vi "Test Parse State.vi"() -> ()   [LabVIEW 2020]
uses:
  <vilib>/regexp/Match Regular Expression.xnode
panel:
  out "Array 2":T1(array[cluster])
  out "Array":T1(array[cluster])
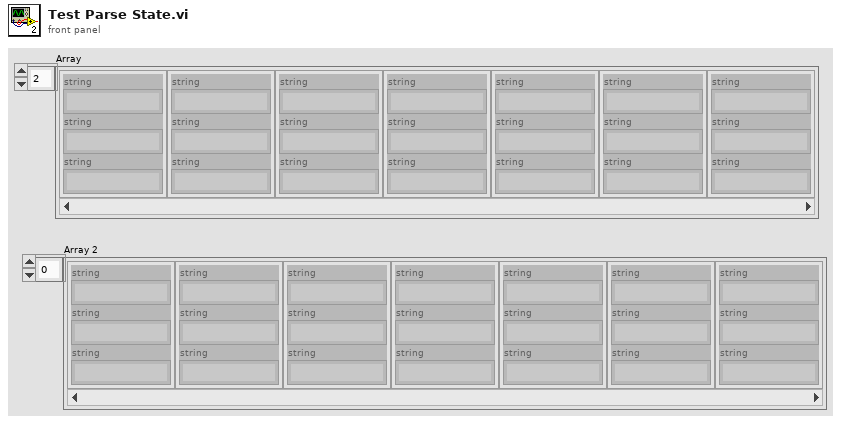
[diagram p1: front panel]
types:
  T1 = cluster{"string":string, "string":string, "string":string}[]
  T2 = cluster{"before match":string, "whole match":string, "after match":string}
  T3 = cluster{"string":string, "string":string, "string":string}
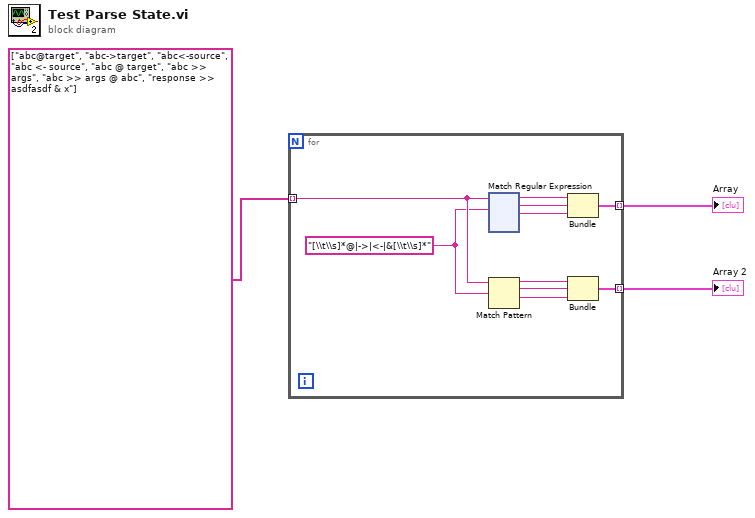
[diagram p0: block diagram]
diagram:
  n1 = for {
    tunnel: string[] ["abc@target", "abc->target", "abc<-source", "abc <- source", "abc @ target", "abc >> args", "abc >> args @ abc", "response >> asdfasdf & x"] ("string") -> [w9] mode=indexing
    tunnel: [w10] -> w2 mode=indexing
    tunnel: [w7] -> w1 mode=indexing
    w8 = "[\\t\\s]*@|->|<-|&[\\t\\s]*" ("regular expression")
    n2 = xnode "Match Regular Expression"("input string"=w9, "regular expression"=w8) -> ("before match"=w13:string, "whole match"=w12:string, "after match"=w11:string)  [unwired: 4 in, 2 out]
    n3 = Match Pattern(string=w9, regular expression=w8) -> (before substring=w6:string, match substring=w5:string, after substring=w4:string)  [unwired: 1 in, 1 out]
    n4 = Bundle("before match"=w13, "whole match"=w12, "after match"=w11) -> (w10:T2)  [unwired: 1 in]
    n5 = Bundle("string"=w6, "string"=w5, "string"=w4) -> (w7:T3)  [unwired: 1 in]
  }
  "Array" <- w2
  "Array 2" <- w1
